vi "RegulatorVARS.vi"() -> ()   [LabVIEW 2015]
panel:
  in  "Regeltakt [ms]":u32=150
  in  "FilmHeightTol [%]":dbl=5.0 format="%#_13g"
  in  "FlowTol [%]":dbl=5.0 format="%#_13g"
  in  "Sens":dbl=0.01 format="%#_13g"
  in  "PID gains":T1={"proportional gain (Kc)"=0.04, "integral time (Ti, min)"=0.02, "derivative time (Td, min)"=0.015} {"derivative time (Td, min)" format="%.3f"; "integral time (Ti, min)" format="%.3f"; "proportional gain (Kc)" format="%.3f"}
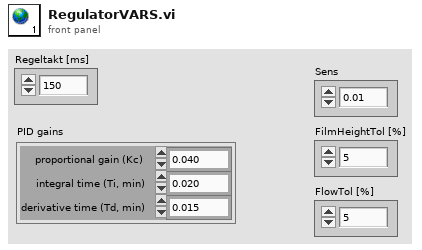
[diagram p1: front panel]
types:
  T1 = cluster{"proportional gain (Kc)":dbl, "integral time (Ti, min)":dbl, "derivative time (Td, min)":dbl}
diagram:
